vi "rvc Vectors to Rotation Matrix.vi"(10 "Vector 2 (A)":dbl[](array[numeric]), 11 "Vector 1 (O)":dbl[](array[numeric])) -> (3 "rotation matrix":T1)   [LabVIEW 2013]
uses:
  <vilib>/Analysis/Matrix/Datatypes/RealMatrix.ctl
  <vilib>/Analysis/_algsub.llb/Vector Norm Type.ctl
  <vilib>/Analysis/baseanly.llb/Unit Vector (DBL).vi
  <vilib>/Analysis/NI_AALPro.lvlib
  <vilib>/Analysis/NI_AALBase.lvlib
  <vilib>/Analysis/Matrix/NI_Matrix.lvlib
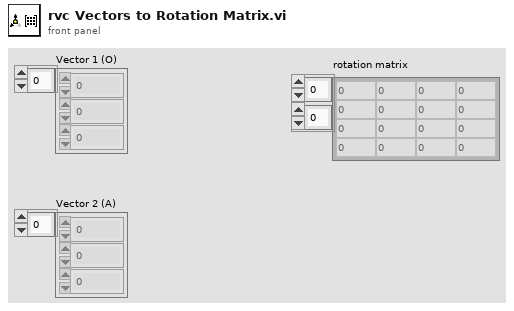
[diagram p1: front panel]
types:
  T1 = typedef "NI_Matrix.lvlib/RealMatrix.ctl" = dbl[][]
  T2 = typedef "NI_AALPro.lvlib/Vector Norm Type.ctl" = u16
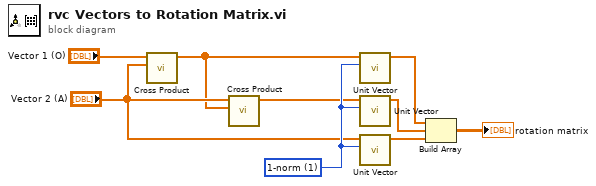
[diagram p0: block diagram]
diagram:
  w6 = T2 1 items=["1-norm"=1, "2-norm"=2, "Inf-norm"=3, "-Inf-norm"=4, "User Defined"=5] ("norm type")
  n1 = call <vilib>:"Cross Product.vi"("B Vector"="Vector 2 (A)", "A Vector"="Vector 1 (O)") -> ("Cross Product"=w1:dbl[])  [unwired: 8 in, 1 out]
  n2 = call <vilib>:"Cross Product.vi"("B Vector"=w1, "A Vector"="Vector 2 (A)") -> ("Cross Product"=w4:dbl[])  [unwired: 8 in, 1 out]
  n3 = call-poly <vilib>:"Unit Vector.vi"("norm type"=w6, "Input Vector"=w1) -> ("Unit Vector"=w5:dbl[])  [unwired: 7 in, 2 out]
  n4 = call-poly <vilib>:"Unit Vector.vi"("norm type"=w6, "Input Vector"=w4) -> ("Unit Vector"=w3:dbl[])  [unwired: 7 in, 2 out]
  n5 = call-poly <vilib>:"Unit Vector.vi"("norm type"=w6, "Input Vector"="Vector 2 (A)") -> ("Unit Vector"=w7:dbl[])  [unwired: 7 in, 2 out]
  n6 = Build Array(w5, w3, w7) -> (→"rotation matrix":T1)
